vi "DPT Air Temperature to Density.vi"(5 "Temp(F)":dbl) -> (6 "Density (lb/ft3)":dbl)   [LabVIEW 2016]
uses:
  <vilib>/gmath/NI_Gmath.lvlib
panel:
  in  "Density":dbl[](array[numeric])=[0.081, 0.08, 0.0766, 0.073, 0.0717, 0.071, 0.0698, 0.0692, 0.0685, 0.0674, 0.0662, 0.0651, 0.064, 0.063, 0.062, 0.061, 0.0601, 0.0592, 0.057, 0.055, 0.0531, 0.0513]
  in  "Temps":dbl[](array[numeric])=[30.0, 40.0, 50.0, 75.0, 85.0, 95.0, 100.0, 105.0, 110.0, 120.0, 130.0, 140.0, 150.0, 160.0, 170.0, 180.0, 190.0, 200.0, 225.0, 250.0, 275.0, 300.0]
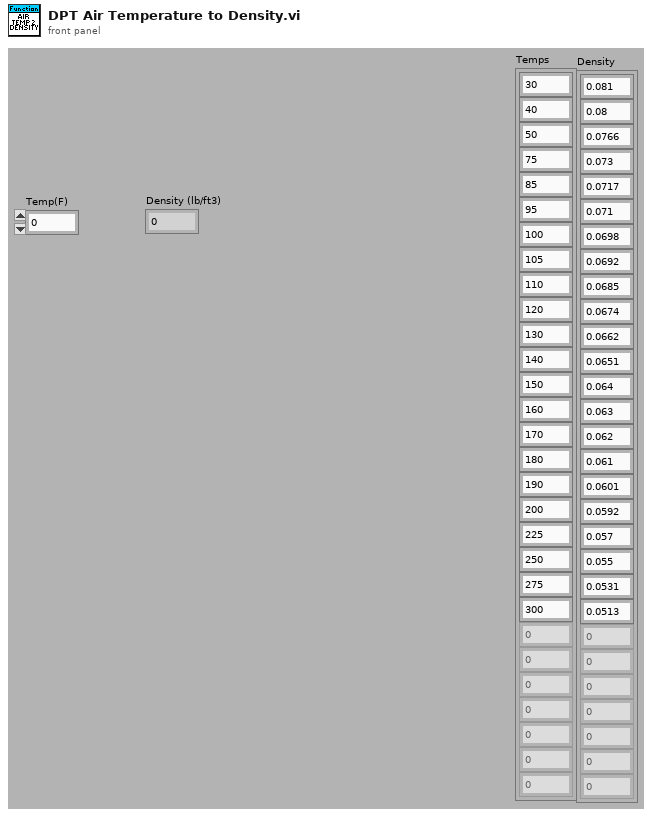
[diagram p1: front panel]
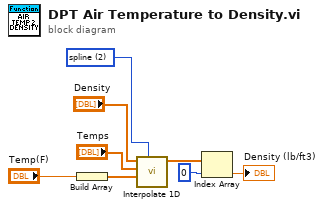
[diagram p0: block diagram]
diagram:
  w8 = 2 items=["nearest", "linear", "spline", "cubic Hermite", "Lagrange"] ("method")
  n1 = Build Array("Temp(F)") -> (w4:dbl[])
  n2 = call <vilib>:"Interpolate 1D.vi"("method"=w8, "xi"=w4, "X"="Temps", "Y"="Density") -> ("yi"=w5:dbl[])  [unwired: 5 in, 2 out]
  n3 = Index Array(array=w5, index=0) -> (element=→"Density (lb/ft3)":dbl)
